vi "FillianProj2.vi"() -> ()   [LabVIEW 2014]
uses:
  <vilib>/ErrorRing/Error Ring.xnode
  <vilib>/Utility/error.llb/Error Cluster From Error Code.vi
panel:
  out "?":bool
  out "?":bool
  out "?":bool
  out "?":bool
  out "?":bool
  out "?":bool
  out "?":bool
  out "?":bool
  out "Voltage too high":bool
  out "Voltage too low":bool
  out "Too cold":bool
  out "Too hot":bool
  in  "Max temp":sgl
  in  "Min temp":sgl
  in  "Min voltage":sgl
  in  "Max voltage":sgl
  out "Minimum voltage":dbl
  out "Max voltage":dbl
  out "Maximum temp":dbl
  out "Minimum temperature":dbl
  out "Mean Temperature":dbl
  out "Mean voltage":dbl
  out "Voltage 2":sgl(graph)
  out "Temperature 2":sgl(graph)
  out "Warnings 2":errorcluster
  out "temp bat timeout":bool
  out "volt bat timeout":bool
  out "volt link timeout":bool
  out "temp link timeout":bool
  out "Link Quality Voltage":sgl
  out "Battery Voltage":sgl
  out "Battery Voltage Temp":sgl
  out "Link Quality Temp":sgl
  in  "stop 2":bool
  # "temperature battery"
  # "voltage battery"
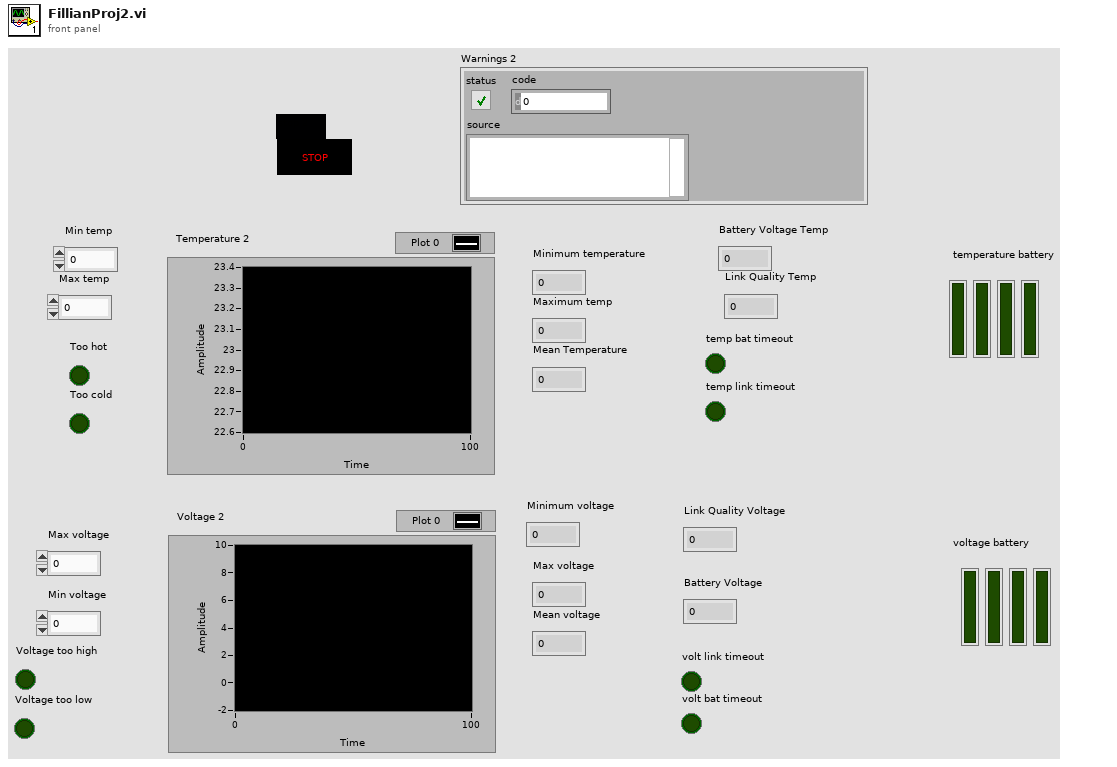
[diagram p1: front panel]
types:
  T1 = enum16{"open", "replace", "create", "open or create", "replace or create", "replace or create with confirmation"}
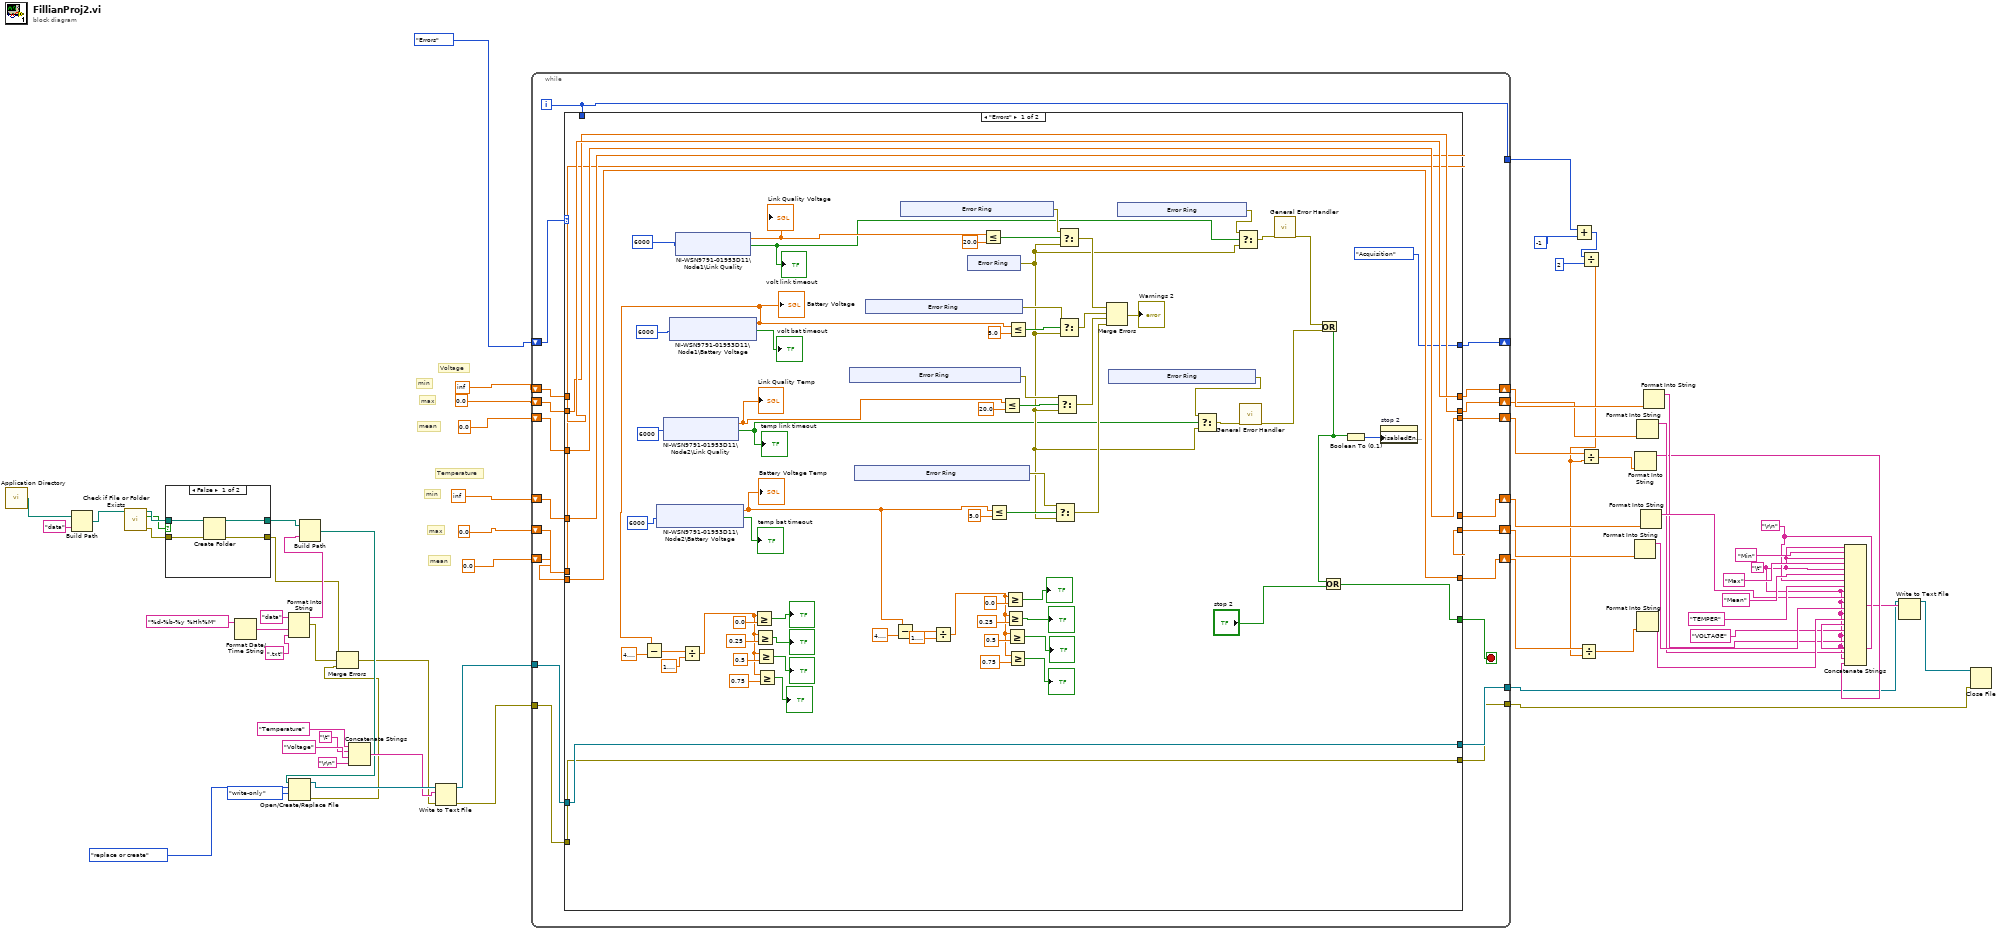
[diagram p0: block diagram]
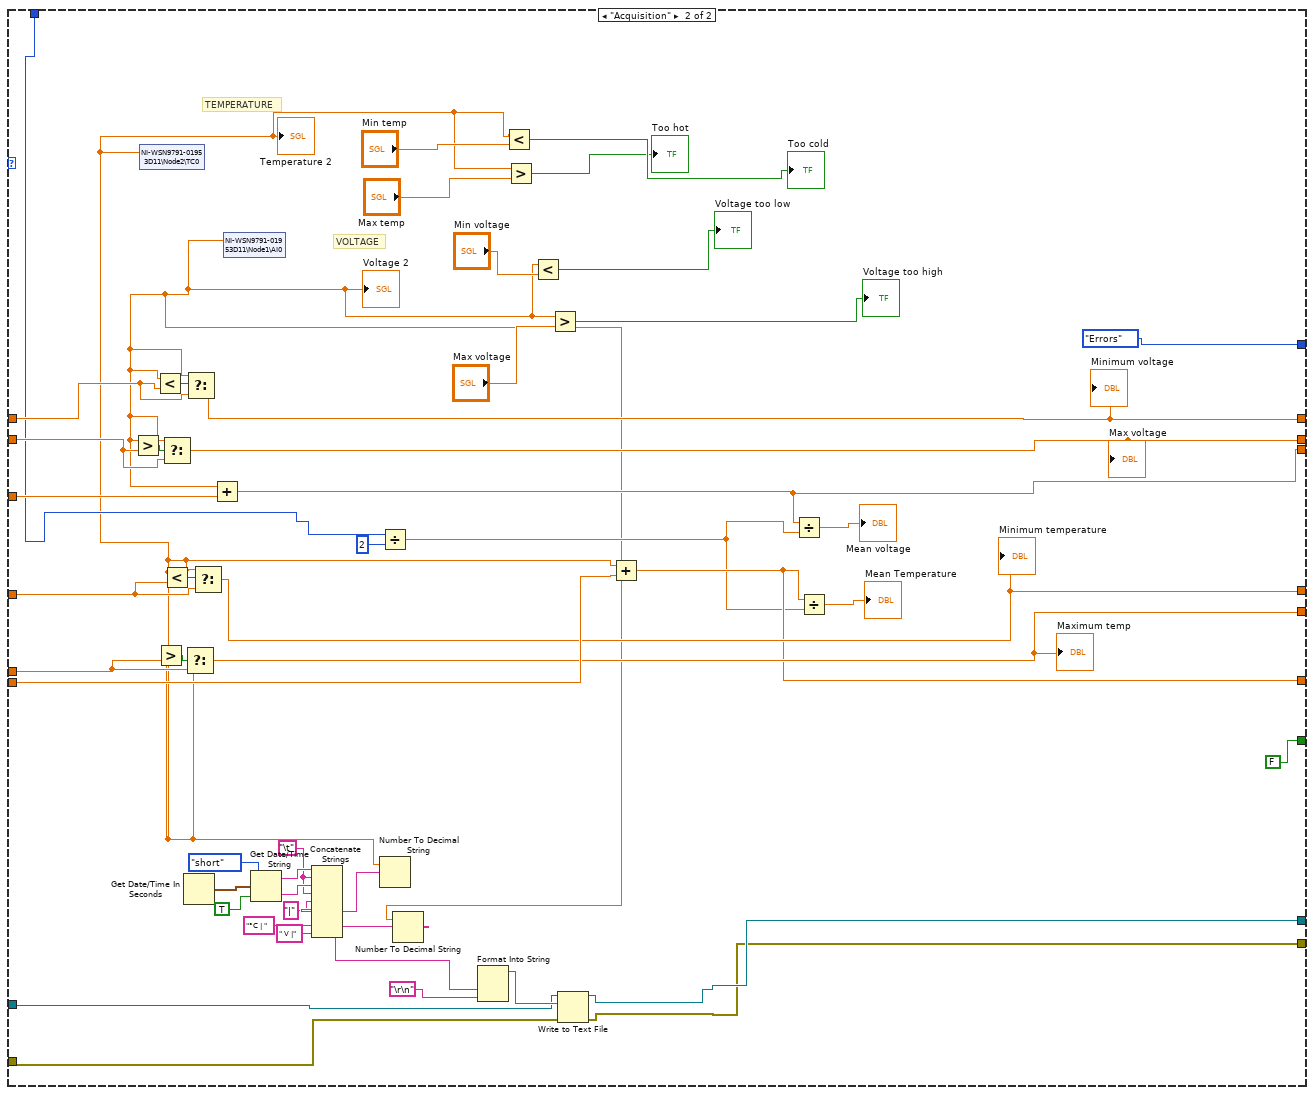
[diagram p3: hidden frame]
diagram:
  w51 = "\r\n"
  w47 = "\t"
  # "max"
  # "mean"
  # "min"
  # "max"
  # "mean"
  # "min"
  # "Voltage"
  # "Temperature"
  n1 = call <vilib>:"Application Directory.vi"() -> ("Application Directory"=w19:path)
  n2 = Build Path(base path=w19, name or relative path="data") -> (appended path=w17:path)
  n3 = call <vilib>:"Check if File or Folder Exists.vi"("path"=w17) -> ("error out"=w15:errorcluster, "file or folder exists?"=w14:bool, "dup path"=w16:path)  [unwired: 8 in]
  n4 = case shown="False" w14 {
    tunnel: w16 -> [w68 w70]
    tunnel: w15 -> [w67 w69]
    tunnel: [w66 w70] -> w13
    tunnel: [w65 w69] -> w5
    frame False {
      n5 = Create Folder(path (use dialog)=w68, error in=w67) -> (created path=w66:path, error out=w65:errorcluster)  [unwired: 1 in, 1 out]
    }
    frame True {
    }
  }
  n6 = Format Date/Time String(time format string (%c)="%d-%b-%y %Hh%M") -> (date/time string=w10:string)  [unwired: 2 in]
  n7 = Format Into String(initial string="data", w10, ".txt") -> (resulting string=w8:string, error out=w6:errorcluster)  [unwired: 2 in]
  n8 = Build Path(base path=w13, name or relative path=w8) -> (appended path=w7:path)
  n9 = Open/Create/Replace File(file path (use dialog)=w7, operation (0:open)=T1."replace or create", access (0:read/write)=enum16{"read/write", "read-only", "write-only"}."write-only") -> (refnum out=w36:refnum<file>, error out=w4:errorcluster)  [unwired: 3 in, 1 out]
  n10 = Merge Errors(w5, w6, w4) -> (w3:errorcluster)
  n11 = Concatenate Strings("Temperature" ("text"), "\t", "Voltage" ("text"), "\r\n") -> (w34:string)
  n12 = Write to Text File(file (use dialog)=w36, text=w34, error in=w3) -> (refnum out=w30:refnum<file>, error out=w29:errorcluster)  [unwired: 1 in, 1 out]
  n13 = while {
    shift-right: [w83] -> w41
    shift-left: inf -> [w89]
    shift-right: [w82] -> w40
    shift-left: 0.0 -> [w88]
    shift-right: [w81] -> w25
    shift-left: 0.0 -> [w87]
    shift-right: [w80] -> w39
    shift-left: inf -> [w86]
    shift-right: [w79] -> w38
    shift-left: 0.0 -> [w85]
    shift-right: [w78] -> w28
    shift-left: 0.0 -> [w84]
    tunnel: [w77] -> w43
    tunnel: [w76] -> w42
    tunnel: w30 -> [w75]
    tunnel: w29 -> [w74]
    tunnel: [w73] -> w22
    shift-right: [w71] -> _
    shift-left: enum16{"Errors", "Acquisition"}."Errors" -> [w72]
    i -> [w73]
    stop <- w90 stop-if-true
    n14 = case shown="\"Errors\"" w72 {
      tunnel: [enum16{"Errors", "Acquisition"}."Acquisition" enum16{"Errors", "Acquisition"}."Errors"] -> w71
      tunnel: [w129 FALSE] -> w90
      tunnel: w89 -> [w127 w240]
      tunnel: w88 -> [w126 w239]
      tunnel: w87 -> [w125 w238]
      tunnel: w86 -> [w124 w237]
      tunnel: w85 -> [w123 w236]
      tunnel: w84 -> [w122 w235]
      tunnel: [w127 w234] -> w83
      tunnel: [w126 w233] -> w82
      tunnel: [w125 w232] -> w81
      tunnel: [w124 w231] -> w80
      tunnel: [w123 w230] -> w79
      tunnel: [w122 w229] -> w78
      tunnel: [w121 w197] -> w77
      tunnel: [w120 w196] -> w76
      tunnel: w75 -> [w121 w226]
      tunnel: w74 -> [w120 w225]
      tunnel: w73 -> [_ w221]
      frame "Errors" {
        n15 = shared-variable "NI-WSN9791-01953D11\\Node2\\Battery Voltage"(6000 ("ms timeout (0)")) -> (w119:sgl, →"temp bat timeout":bool)  [unwired: 1 in, 1 out]
        "Battery Voltage Temp" <- w119
        n16 = shared-variable "NI-WSN9791-01953D11\\Node2\\Link Quality"(6000 ("ms timeout (0)")) -> (w142:sgl, w91:bool)  [unwired: 1 in, 1 out]
        "Link Quality Temp" <- w142
        "temp link timeout" <- w91
        n17 = shared-variable "NI-WSN9791-01953D11\\Node1\\Battery Voltage"(6000 ("ms timeout (0)")) -> (w94:sgl, →"volt bat timeout":bool)  [unwired: 1 in, 1 out]
        "Battery Voltage" <- w94
        n18 = Subtract(x=w94, y=sgl 4.8) -> (x-y=w105:sgl)
        n19 = shared-variable "NI-WSN9791-01953D11\\Node1\\Link Quality"(6000 ("ms timeout (0)")) -> (w146:sgl, w137:bool)  [unwired: 1 in, 1 out]
        "Link Quality Voltage" <- w146
        "volt link timeout" <- w137
        n20 = Divide(x=w105, y=sgl 1.4) -> (x/y=w99:sgl)
        n21 = Greater Or Equal?(x=w99, y=0.0) -> (x >= y?=→"?":bool)
        n22 = Greater Or Equal?(x=w99, y=0.25) -> (x >= y?=→"?":bool)
        n23 = Greater Or Equal?(x=w99, y=0.5) -> (x >= y?=→"?":bool)
        n24 = Greater Or Equal?(x=w99, y=0.75) -> (x >= y?=→"?":bool)
        n25 = xnode "Error Ring"() -> ("error out"=w160:errorcluster)
        n26 = xnode "Error Ring"() -> ("error out"=w148:errorcluster)
        n27 = xnode "Error Ring"() -> ("error out"=w155:errorcluster)
        n28 = Subtract(x=w119, y=sgl 4.8) -> (x-y=w117:sgl)
        n29 = xnode "Error Ring"() -> ("error out"=w157:errorcluster)
        n30 = Divide(x=w117, y=sgl 1.4) -> (x/y=w111:sgl)
        n31 = xnode "Error Ring"() -> ("error out"=w135:errorcluster)
        n32 = Less Or Equal?(x=w146, y=sgl 20.0) -> (x <= y?=w158:bool)
        n33 = Less Or Equal?(x=w119, y=sgl 5.0) -> (x <= y?=w149:bool)
        n34 = Less Or Equal?(x=w142, y=sgl 20.0) -> (x <= y?=w161:bool)
        n35 = Greater Or Equal?(x=w111, y=0.0) -> (x >= y?=→"?":bool)
        n36 = Greater Or Equal?(x=w111, y=0.25) -> (x >= y?=→"?":bool)
        n37 = Greater Or Equal?(x=w111, y=0.5) -> (x >= y?=→"?":bool)
        n38 = Greater Or Equal?(x=w111, y=0.75) -> (x >= y?=→"?":bool)
        n39 = Less Or Equal?(x=w94, y=sgl 5.0) -> (x <= y?=w156:bool)
        n40 = Select(t=w148, s=w149, f=w135) -> (s? t:f=w147:errorcluster)
        n41 = Select(t=w160, s=w161, f=w135) -> (s? t:f=w151:errorcluster)
        n42 = Select(t=w157, s=w158, f=w135) -> (s? t:f=w153:errorcluster)
        n43 = Select(t=w155, s=w156, f=w135) -> (s? t:f=w154:errorcluster)
        n44 = Merge Errors(w153, w154, w151, w147) -> (→"Warnings 2":errorcluster)
        n45 = xnode "Error Ring"() -> ("error out"=w136:errorcluster)
        n46 = xnode "Error Ring"() -> ("error out"=w138:errorcluster)
        n47 = Select(t=w136, s=w91, f=w135) -> (s? t:f=w133:errorcluster)
        n48 = Select(t=w138, s=w137, f=w135) -> (s? t:f=w134:errorcluster)
        n49 = call <vilib>:"General Error Handler.vi"("error in (no error)"=w133) -> ("error out"=w131:errorcluster)  [unwired: 10 in, 4 out]
        n50 = call <vilib>:"General Error Handler.vi"("error in (no error)"=w134) -> ("error out"=w132:errorcluster)  [unwired: 10 in, 4 out]
        n51 = Or(x=w132, y=w131) -> (x .or. y?=w128:bool)
        n52 = Or(x=w128, y="stop 2") -> (x .or. y?=w129:bool)
        n53 = Boolean To (0,1)(Boolean=w128) -> (0, 1=w130:i16)
        n54 = property on="stop 2" class="Bool"("DisabledEnum"=w130) -> ()  [unwired: 2 in, 2 out]
      }
      frame "Acquisition" {
        w207 = "\t"
        # "VOLTAGE"
        # "TEMPERATURE"
        n55 = shared-variable "NI-WSN9791-01953D11\\Node2\\TC0"() -> (w206:sgl)  [unwired: 1 in, 1 out]
        "Temperature 2" <- w206
        n56 = Greater?(x=w206, y=w236) -> (0:w242:bool)
        n57 = Less?(x=w206, y=w237) -> (x < y?=w243:bool)
        n58 = Get Date/Time In Seconds() -> (seconds since 1Jan1904=w212:timestamp)
        n59 = Select(t=w206, s=w242, f=w236) -> (s? t:f=w230:dbl)
        "Maximum temp" <- w230
        n60 = Select(t=w206, s=w243, f=w237) -> (s? t:f=w231:dbl)
        "Minimum temperature" <- w231
        n61 = shared-variable "NI-WSN9791-01953D11\\Node1\\AI0"() -> (w202:sgl)  [unwired: 1 in, 1 out]
        "Voltage 2" <- w202
        n62 = Greater?(x=w202, y=w239) -> (0:w245:bool)
        n63 = Less?(x=w202, y=w240) -> (x < y?=w244:bool)
        n64 = Select(t=w202, s=w245, f=w239) -> (s? t:f=w233:dbl)
        "Max voltage" <- w233
        n65 = Select(t=w202, s=w244, f=w240) -> (s? t:f=w234:dbl)
        "Minimum voltage" <- w234
        n66 = Add(x=w202, y=w238) -> (x+y=w232:dbl)
        n67 = Get Date/Time String(date format (0)=enum16{"short", "long", "abbreviated"}."short", seconds (now)=w212, want seconds? (F)=TRUE) -> (date string=w209:string, time string=w208:string)
        n68 = Divide(x=w221, y=2) -> (x/y=w223:dbl)
        n69 = Number To Decimal String(number=w206) -> (decimal integer string=w205:string)  [unwired: 1 in]
        n70 = Number To Decimal String(number=w202) -> (decimal integer string=w201:string)  [unwired: 1 in]
        n71 = Concatenate Strings(w209, w207, w208, w207, "|" ("string"), w205, "°C | " ("string"), w201, " V |" ("string")) -> (w198:string)
        n72 = Format Into String(w198, "\r\n") -> (resulting string=w241:string)  [unwired: 3 in, 1 out]
        n73 = Less?(x=w206, y="Min temp") -> (x < y?=→"Too cold":bool)
        n74 = Greater?(x=w206, y="Max temp") -> (0:→"Too hot":bool)
        n75 = Less?(x=w202, y="Min voltage") -> (x < y?=→"Voltage too low":bool)
        n76 = Greater?(x=w202, y="Max voltage") -> (0:→"Voltage too high":bool)
        n77 = Write to Text File(file (use dialog)=w226, text=w241, error in=w225) -> (refnum out=w197:refnum<file>, error out=w196:errorcluster)  [unwired: 1 in, 1 out]
        n78 = Add(x=w206, y=w235) -> (x+y=w229:dbl)
        n79 = Divide(x=w232, y=w223) -> (x/y=→"Mean voltage":dbl)
        n80 = Divide(x=w229, y=w223) -> (x/y=→"Mean Temperature":dbl)
      }
    }
  }
  n81 = Add(x=w22, y=-1) -> (x+y=w23:i32)
  n82 = Divide(x=w23, y=2) -> (x/y=w20:dbl)
  n83 = Divide(x=w28, y=w20) -> (x/y=w26:dbl)
  n84 = Divide(x=w25, y=w20) -> (x/y=w24:dbl)
  n85 = Format Into String(w38) -> (resulting string=w53:string)  [unwired: 3 in, 1 out]
  n86 = Format Into String(w24) -> (resulting string=w46:string)  [unwired: 3 in, 1 out]
  n87 = Format Into String(w40) -> (resulting string=w48:string)  [unwired: 3 in, 1 out]
  n88 = Format Into String(w26) -> (resulting string=w52:string)  [unwired: 3 in, 1 out]
  n89 = Format Into String(w39) -> (resulting string=w54:string)  [unwired: 3 in, 1 out]
  n90 = Format Into String(w41) -> (resulting string=w49:string)  [unwired: 3 in, 1 out]
  n91 = Concatenate Strings(w47, "Min", w47, "Max", w47, "Mean", w51, "TEMPER", w47, w54, w47, w53, w47, w52, w51, "VOLTAGE", w47, w49, w47, w48, w47, w46) -> (w45:string)
  n92 = Write to Text File(file (use dialog)=w43, text=w45) -> (refnum out=w44:refnum<file>)  [unwired: 2 in, 2 out]
  n93 = Close File(refnum=w44, error in=w42) -> ()  [unwired: 2 out]
